vi "Maj pixels.vi"(10 "Pixel  B":cluster{"Rouge : ":u8, "Vert :":u8, "Bleu :":u8}, 11 "Pixel H":cluster{"Rouge : ":u8, "Vert :":u8, "Bleu :":u8}) -> (2 "Oct Mx P1 2":u8, 3 "Oct Mx P1":u8)   [LabVIEW 2014]
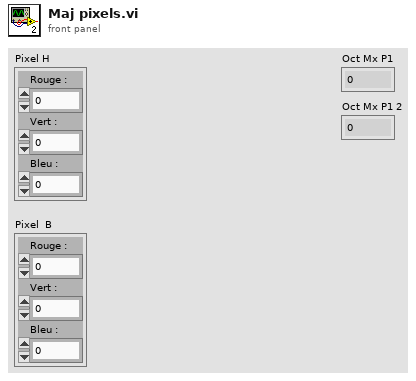
[diagram p1: front panel]
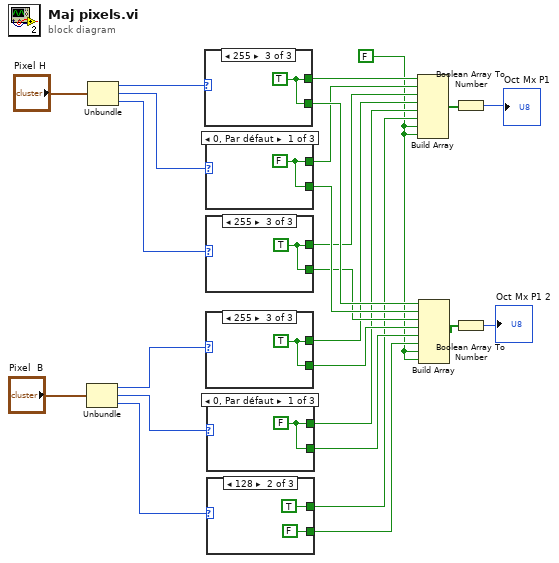
[diagram p0: block diagram]
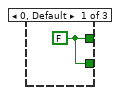
[diagram p2: hidden frame]
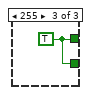
[diagram p3: hidden frame]
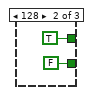
[diagram p4: hidden frame]
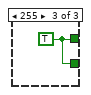
[diagram p5: hidden frame]
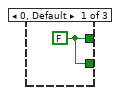
[diagram p6: hidden frame]
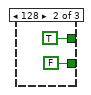
[diagram p7: hidden frame]
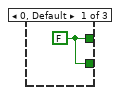
[diagram p8: hidden frame]
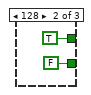
[diagram p9: hidden frame]
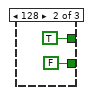
[diagram p10: hidden frame]
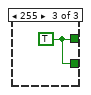
[diagram p11: hidden frame]
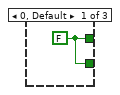
[diagram p12: hidden frame]
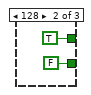
[diagram p13: hidden frame]
diagram:
  w5 = FALSE
  n1 = Unbundle("Pixel  B") -> ("Rouge :"=w14:u8, "Vert :"=w13:u8, "Bleu :"=w12:u8)
  n2 = Unbundle("Pixel H") -> ("Rouge :"=w23:u8, "Vert :"=w20:u8, "Bleu :"=w19:u8)
  n3 = case shown="255" w23 {
    tunnel: [w26 TRUE w29] -> w22
    tunnel: [w26 FALSE w29] -> w21
    frame 0, Default {
      w26 = FALSE
    }
    frame 128 {
    }
    frame 255 {
      w29 = TRUE
    }
  }
  n4 = case shown="0, Par défaut" w20 {
    tunnel: [w30 TRUE w33] -> w18
    tunnel: [w30 FALSE w33] -> w17
    frame 0, Default {
      w30 = FALSE
    }
    frame 128 {
    }
    frame 255 {
      w33 = TRUE
    }
  }
  n5 = case shown="255" w19 {
    tunnel: [w34 TRUE w37] -> w16
    tunnel: [w34 FALSE w37] -> w15
    frame 0, Default {
      w34 = FALSE
    }
    frame 128 {
    }
    frame 255 {
      w37 = TRUE
    }
  }
  n6 = case shown="255" w14 {
    tunnel: [w38 TRUE w41] -> w11
    tunnel: [w38 FALSE w41] -> w10
    frame 0, Default {
      w38 = FALSE
    }
    frame 128 {
    }
    frame 255 {
      w41 = TRUE
    }
  }
  n7 = case shown="0, Par défaut" w13 {
    tunnel: [w42 TRUE w45] -> w9
    tunnel: [w42 FALSE w45] -> w8
    frame 0, Default {
      w42 = FALSE
    }
    frame 128 {
    }
    frame 255 {
      w45 = TRUE
    }
  }
  n8 = case shown="128" w12 {
    tunnel: [w46 TRUE w49] -> w7
    tunnel: [w46 FALSE w49] -> w6
    frame 0, Default {
      w46 = FALSE
    }
    frame 128 {
    }
    frame 255 {
      w49 = TRUE
    }
  }
  n9 = Build Array(w22, w18, w16, w11, w9, w7, w5, w5) -> (w4:bool[])
  n10 = Build Array(w21, w17, w15, w10, w8, w6, w5, w5) -> (w2:bool[])
  n11 = Boolean Array To Number ("Tableau de booléens en nombre")(Boolean array=w4) -> (number=→"Oct Mx P1":u8)
  n12 = Boolean Array To Number ("Tableau de booléens en nombre")(Boolean array=w2) -> (number=→"Oct Mx P1 2":u8)
